vi "Sensors Global.vi"() -> ()   [LabVIEW 2018]
panel:
  out "Panel Sensor 3":bool
  out "HatchLimit Switch 2":bool
  out "Panel Sensor 2":bool
  out "HatchLimit Switch":bool
  out "HatchOpened":bool
  out "HatchExtended":bool
  out "Panel Sensor":bool
  out "Cargo Sensor":bool
  out "HAB Retracting limit":bool
  out "HAB Extending limit":bool
  in  "Calc Time difference":bool
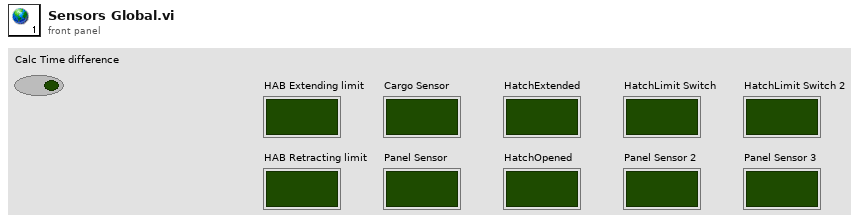
[diagram p1: front panel]
diagram:
